vi "LEBITplc.ReadoutSetra.vi"(0 "i ref in":refnum<vi>, 5 "error in":errorcluster) -> (14 "i ref out":refnum<vi>, 19 "error IO":errorcluster)   [LabVIEW 2014, in "LEBITplc.lvlib"]
uses:
  LEBITplc.lvlib
  <vilib>/Utility/error.llb/whitespace.ctl
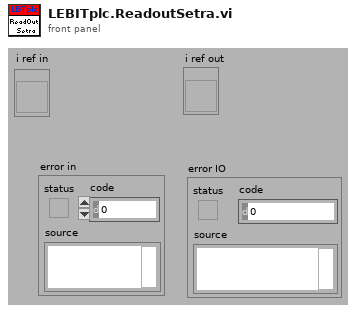
[diagram p1: front panel]
types:
  T1 = enum16{"Read", "Write", "ReadWrite", "BufferedRead", "BufferedReadWrite"}
  T2 = typedef "whitespace.ctl" = u16
  T3 = typedef "LEBITplc.lvlib/LEBITplc.i attribute.ctl" = cluster{"LLFLocation":string, "SetFileLocation":string, "nickNames":string[], "setValuePLCServiceID":i32[], "GUIServiceID":i32[], "monValuePLC":string[], "SetValueServiceID":i32[], "MonValueServiceID":i32[], "SetValue":dbl[][], "SetValueMin":dbl[], "SetValueMax":dbl[], "SetValueInfoServiceID":i32[], "GUINames":string[], "ListOfBases":string[], "Scale":dbl[], "Offset":dbl[], "setValuePLC":string[], "BaseName":string[], "ScaleServiceID":i32[], "OffsetServiceID":i32[], "AllPLCValues":string[], "CondSpecialArray":string[][], "CondSpecialIndex":i32[], "CondSpecialMonValue":dbl[], "RecentlyChanged":i32[], "SetFileLocationID":i32, "Dependent-Monitors":string[][], "LastLoadedFiles":string[], "IonGuideCalibLocation":string, "Monitor Dependent":string[], "Special":string[], "PLC?":bool[], "Start Date":string, "ListOfBasesServiceID":i32, "SETRA VISA resource":refnum<visa-resource-name>}
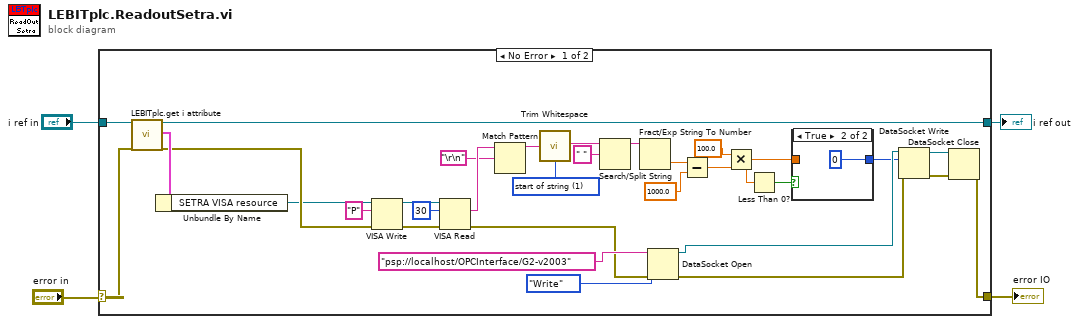
[diagram p0: block diagram]
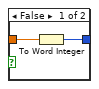
[diagram p2: hidden frame]
diagram:
  n1 = case shown="No Error" "error in" {
    selector: "error in" -> [w10 w41]
    tunnel: [w15 w41] -> w3
    tunnel: "i ref in" -> [w11 w40]
    tunnel: [w9 w40] -> w1
    frame No Error {
      w30 = T2 1 items=["both", "start of string", "end of string"] ("location (both)")
      n2 = call "LEBITplc.get i attribute.vi"("i ref in"=w11, "error in (no error)"=w10) -> ("i ref out"=w9:refnum<vi>, "i attribute"=w8:T3, "error out"=w7:errorcluster)  [unwired: 15 in]
      n3 = Unbundle By Name(w8) -> ("SETRA VISA resource"=w6:refnum<visa-resource-name>)
      n4 = VISA Write(VISA resource name=w6, write buffer="P", error in (no error)=w7) -> (VISA resource name out=w34:refnum<visa-resource-name>, error out=w35:errorcluster)  [unwired: 1 out]
      n5 = VISA Read(VISA resource name=w34, byte count=u32 30, error in (no error)=w35) -> (read buffer=w32:string, error out=w5:errorcluster)  [unwired: 2 out]
      n6 = Match Pattern(string=w32, regular expression="\r\n") -> (before substring=w26:string)  [unwired: 1 in, 3 out]
      n7 = call <vilib>:"Trim Whitespace.vi"("string"=w26, "location (both)"=w30) -> ("trimmed string"=w29:string)
      n8 = Search/Split String(string=w29, search string/char (-)=" ") -> (substring before match=w27:string)  [unwired: 1 in, 2 out]
      n9 = Fract/Exp String To Number(string=w27) -> (number=w25:dbl)  [unwired: 3 in, 1 out]
      n10 = DataSocket Open(8:w5, 10:T1."Write" ("mode"), 11:"psp://localhost/OPCInterface/G2-v2003" ("connection in")) -> (0:w17:errorcluster, 3:w19:refnum<k13>)  [unwired: 1 in]
      n11 = Subtract(x=w25, y=1000.0) -> (x-y=w23:dbl)
      n12 = Multiply(x=100.0, y=w23) -> (x*y=w12:dbl)
      n13 = Less Than 0?(x=w12) -> (x < 0?=w14:bool)
      n14 = case shown="True" w14 {
        tunnel: [w38 i16 0 ("number")] -> w13
        tunnel: w12 -> [w37 _]
        frame False {
          n15 = To Word Integer(number=w37) -> (16bit integer=w38:i16)
        }
        frame True {
        }
      }
      n16 = DataSocket Write(8:w17, 10:w13, 11:w19) -> (0:w16:errorcluster, 3:w18:refnum<k13>)  [unwired: 1 in, 1 out]
      n17 = DataSocket Close(8:w16, 11:w18) -> (0:w15:errorcluster)  [unwired: 1 in, 1 out]
    }
    frame Error {
    }
  }
  "error IO" <- w3
  "i ref out" <- w1
